vi "List.vi"(8 "error in (no error)":errorcluster) -> (0 "error out":errorcluster, 3 "All Timers":T1(array[cluster]))   [LabVIEW 2021, in "QueueTimer.lvlib"]
doc: "List all queue timers in memory. This groups the queue timers by queue reference."
uses:
  QueueTimer.lvlib
  <vilib>/Utility/miscctls.llb/LVMapReplaceAction.ctl
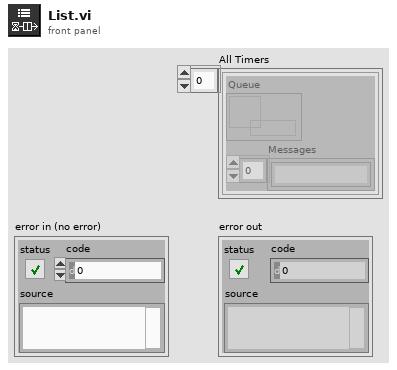
[diagram p1: front panel]
types:
  T1 = cluster{"Queue":refnum<queue>, "Messages":string[]}[]
  T2 = typedef "LVMapReplaceAction.ctl" = enum32{"Modify Entry only if found", "Add or Modify Entry", "Delete Entry"}
  T3 = map{cluster{"Queue":refnum<queue>, "Message":string}, cluster{"Emit":refnum<queue>, "Time":refnum<data-value>, "Daemon":refnum<vi>}}
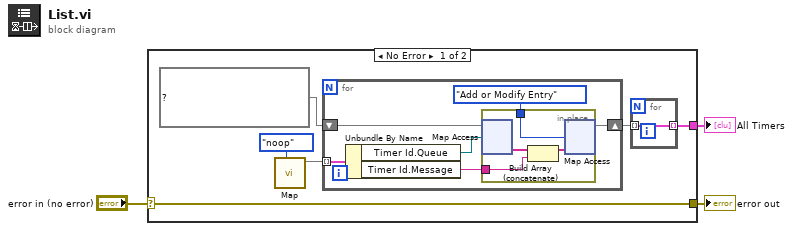
[diagram p0: block diagram]
diagram:
  n1 = case shown="No Error" "error in (no error)" {
    selector: "error in (no error)" -> [w4 w21]
    tunnel: [w5 _] -> w3
    tunnel: [w4 w21] -> w2
    frame No Error {
      n2 = call "Map.vi"("Action"=enum8{"noop", "get", "set", "pop"}."noop") -> ("Timers Map"=w8:T3)  [unwired: 8 in, 2 out]
      n3 = for {
        tunnel: w8 -> [w15] mode=indexing
        shift-right: [w10] -> w6
        shift-left: map{refnum<queue>, string[]} {} ("Map") -> [w14]
        n4 = Unbundle By Name(w15) -> ("Timer Id.Queue"=w12:refnum<queue>, "Timer Id.Message"=w11:string)
        n5 = in-place {
          in-place-border: LVMapReplaceAction."Add or Modify Entry" ("action") -> [w19]
          in-place-border: w11 -> [w16]
          n6 = in-place-map #1(w14, w12) -> (w18:string[])  [unwired: 1 in, 1 out]
          n7 = Build Array (concatenate)(w18, w16) -> (w17:string[])
          n8 = in-place-map #1(w17, w19) -> (w10:map{refnum<queue>, string[]})  [unwired: 2 out]
        }
      }
      n9 = for {
        tunnel: w6 -> [w20] mode=indexing
        tunnel: [w20] -> w5 mode=indexing
      }
    }
    frame Error {
    }
  }
  "error out" <- w2
  "All Timers" <- w3
